vi "Send Create Channel Arbitrary Waveform [ACH].vi"(7 "Message Priority (Normal)":T1=enum."Normal", 8 "error in (no error)":errorcluster, 9 "Channel Name (\"\")":string="CHANNEL1" caption="channel name (\"CHANNEL1\")", 10 "waveform data array (empty)":dbl[](array[numeric]) format="%.3f", 11 "Message Enqueuer":refnum<class "Message Enqueuer.lvclass">) -> (0 "error out":errorcluster, 3 "Message Enqueuer out":refnum<class "Message Enqueuer.lvclass">)   [LabVIEW 2013, in "CS++Fgen.lvlib" / "Create Channel Arbitrary Waveform [ACH] Msg.lvclass"]
doc: "This VI sends the message to an actor."
uses:
  Create Channel Arbitrary Waveform [ACH] Msg.lvclass
  <vilib>/ActorFramework/Message Enqueuer/Message Enqueuer.lvclass
  <vilib>/ActorFramework/Message Enqueuer/Message Priority.ctl
  Create Channel Arbitrary Waveform [ACH] Msg.lvclass/Create Channel Arbitrary Waveform [ACH] Msg.ctl
  <vilib>/ActorFramework/Message Enqueuer/Message Enqueuer.lvclass/Message Enqueuer.ctl
  <vilib>/ActorFramework/Message Priority Queue/Priority Enqueue.vi
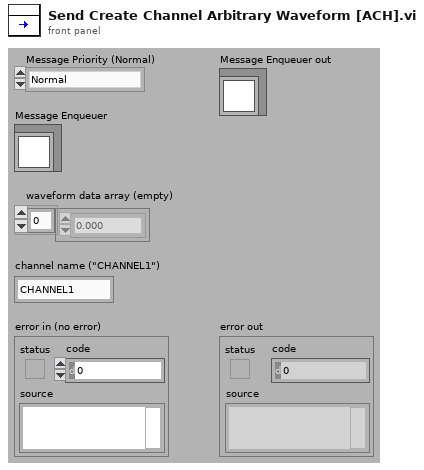
[diagram p1: front panel]
types:
  T1 = typedef "Actor Framework.lvlib/Message Enqueuer.lvclass/Message Priority.ctl" = enum16{"Low", "Normal", "High"}
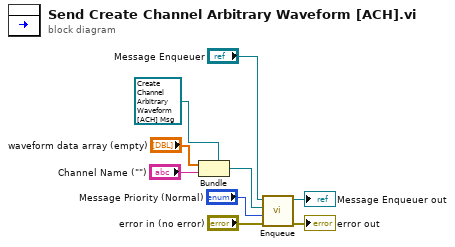
[diagram p0: block diagram]
diagram:
  n1 = Bundle(cluster=refnum<class "Create Channel Arbitrary Waveform [ACH] Msg.lvclass"> refnum ("Object"), "waveform data array (empty)", "Channel Name (\"\")") -> (w5:refnum<class "Create Channel Arbitrary Waveform [ACH] Msg.lvclass">)
  n2 = call <vilib>:"Enqueue.vi"("error in (no error)"="error in (no error)", "Message Priority (Normal)"="Message Priority (Normal)", "Message"=w5, "Message Enqueuer in"="Message Enqueuer") -> ("error out"=→"error out":errorcluster, "Message Enqueuer out"=→"Message Enqueuer out":refnum<class "Message Enqueuer.lvclass">)  [unwired: 6 in]
